vi "CR test.vi"() -> ()   [LabVIEW 2021]
uses:
  Data Model/ELAN Data Model/Type Definitions/Value full.ctl
  Data Unit/ELAN PC Data Unit/Elan units.ctl
  Data Unit/ELAN PC Data Unit/Elan measured variable.ctl
  Data Unit/ELAN PC Data Unit/Elan channel state.ctl
  enums/main_prog_state.ctl
  enums/init_state.ctl
  Master CR.lvclass
  Param/TCP Param/TCP Param.lvclass
  D:/my_projects/projects/Algorithms/Labview/21/Master CR/Param/Param.lvclass
  Master CR.lvclass/Master CR.ctl
  Param/Param.lvclass/Param.ctl
  Param/TCP Param/TCP Param.lvclass/TCP Param.ctl
  <vilib>/Platform/TimedLoop/XDataNode/timing_clust.ctl
  <vilib>/Platform/TimedLoop/XDataNode/nitl_modes.ctl
  <vilib>/Platform/TimedLoop/XDataNode/wakeup.ctl
  enums/close_state.ctl
  Data/Data Model/Read Data Model.vi
  <vilib>/Platform/TimedLoop/XDataNode/XDataNode.xnode
  Modbus_v121c/Data Model/Device Data Model.lvclass
  <vilib>/Platform/TimedLoop/XDataNode/XDNodeRunTimeDep.lvlib
  enums/Param_MB test.lvlib
  Param/Param.lvclass
  Data Model/ELAN Data Model/ELAN Data Model.lvclass
  Data Unit/ELAN PC Data Unit/ELAN PDU.lvclass
panel:
  out "PM3112":dbl[][](array[numeric])
  out "Values":T1[][](array[typedef]) {"Value"."Value" format="%#_6f"}
  in  "Write":bool
  in  "Read":bool
  out "connects":bool[](array[boolean])
  out "DI":bool[][](array[boolean])
  out "AI":u16[][](array[numeric])
  in  "DO":bool[][](array[boolean])
  in  "AOint":u16[][](array[numeric])
  out "comm error":errorcluster
  out "initialise error":errorcluster
  in  "EP_on":bool
  in  "tick":i64=100 caption="Время цикла основной программы" min=5 max=500 step=1
  in  "stop":bool
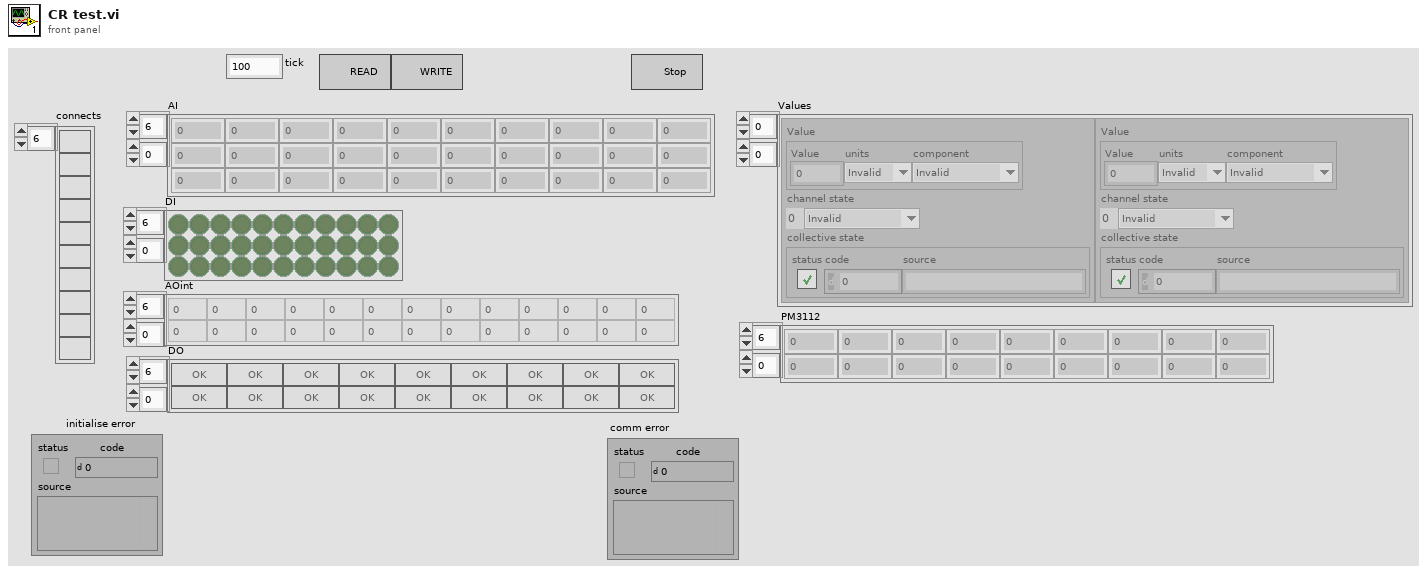
[diagram p1: front panel]
types:
  T1 = typedef "ELAN Data Model.lvclass/Value full.ctl" = cluster{"Value":cluster{"Value":sgl, "units":T2, "component":T3}, "channel state":T4, "collective state":errorcluster}
  T2 = typedef "ELAN PDU.lvclass/Elan units.ctl" = enum16{"Invalid", "no dimension", "ppm", "ppb", "vpm", "ppm C1", "ppm C3", "ppm C6", "mg C/m3", "mg/m3", "%", "% vol", "% of measuring range", "% saturation", "%/°C", "%/K", "% weight", "mV/pH", "mV/mbar", "nA/mbar", "S/m", "S/cm", "mS/m", "mS/cm", "мS/m", "мS/cm", "S", "min", "H", "Pa", "MA", "uV", "MV", "V", "mbar", "hPa", "Ml/min", "kOhm", "MOhm", "S1", "°C", "Hz", "pH", "ug/l", "mg/l", "l/min", "uA", "mg/dm3", "kPa", "kOhm*cm", "MOhm*cm", "°", "1/min", "1/m", "g/m3", "g/l", "% Vol C"}
  T3 = typedef "ELAN PDU.lvclass/Elan measured variable.ctl" = enum16{"Invalid", "no component", "CO", "CO2", "CH4 (Methan)", "C6H14 (Hexan)", "SO2", "NO", "NO2", "CHClF2 (R22)", "C3H8 (Propan)", "C4H10 (Butan)", "O2", "C5H12 (Pentan)", "CnHm (THC)", "P (process pressure)", "pH", "T (temperature)", "C2H4 (Ethen)", "C2H2 (Ethin)", "C3H6 (Propen)", "C4H6", "C4H8", "C2H6", "NH3 (Ammoniak)", "N2O", "C6H6 (Benzol)", "SF6", "CH3OH (Methanol)", "C2H5OH (Ethanol)", "CH2Cl2", "C2H4Cl2", "CH3Cl", "C2H4O", "H2O (water vapor)", "G/l (conductivity)", "C", "S", "N", "CF4", "COCl2 (phosgene)", "CHF3 (R23)", "C2F6 (R116)", "------ (self defined component)", "C2H3Cl", "H2 (Hydrogen)", "Ar", "He", "Cl2", "N2"}
  T4 = typedef "ELAN PDU.lvclass/Elan channel state.ctl" = enum16{"Invalid", "Warm-up", "Pause", "Standby", "Measure", "Zero calibration", "Adjust component slope", "Not yet defined1", "Adjust curve dip", "Adjust linearization sensitivity", "Adjust temperature compensation", "Adjust pressure compensation", "Adjust linearization zero", "Not yet defined2", "Autocal", "Adjust phase", "Zero calibration of O2 sensor", "Synchronous zero calibration", "Purging for synchronous zero calibration", "Adjust analog output", "Adjust analog input", "Autocal check"}
  T5 = cluster{"conn_timeout":i32, "reconn_timeout":i32, "N attempt max":i32, "t_reset_TTL":i32, "write_timeout":i32, "read_timeout":i32, "period":i32}[]
  T6 = cluster{"Remote IP Address":string, "Remote Port":u16}[]
  T7 = typedef "Param_MB test.lvlib/init_state.ctl" = enum16{"Init Data", "Init TMPs", "Init system DB", "Init data DB", "Read Enums", "Init arrays", "Init KFM", "Init Param", "Init AI param", "Init DI param", "Init AO param", "Init DO param", "Init ALR param", "Init save progs", "Read OPC param", "Init Shared Variables", "Init regulators", "Init heaters", "Init Y defs", "Exit"}
  T8 = typedef "Param_MB test.lvlib/main_prog_state.ctl" = enum16{"Read_AI_Param", "Read_DI_Param", "Read_AO_Param", "Read_DO_Param", "Read_ALR_ON_OFF", "Read_ALR_Param", "Read_Param", "Read_REG_Param", "Timers", "AI", "DI", "SendAItoScada", "SendDItoScada", "Alarms", "SendAItoDB", "SendDItoDB", "SendALRtoDB", "Messages", "Controls", "Control HT1", "QN_control", "QN", "QN_state", "Control EB3", "Outputs", "Exit"}
  T9 = cluster{"KFM":string[], "PAR":string[], "AI":string[], "DI":string[], "DI_fast":string[], "AO":string[], "Regs":string[], "DO":string[], "ALR":string[], "System":string[]}
  T10 = cluster{"Enums":cluster{"KFM":string[], "PAR":string[], "AI":string[], "DI":string[], "DI_fast":string[], "AO":string[], "Regs":string[], "DO":string[], "ALR":string[], "System":string[]}, "MBs":refnum<class "Master CR.lvclass">[]}
  T11 = cluster{"current time":timestamp, "Timer_1s":bool, "Timer_10s":bool, "Timer_1day":bool}
  T12 = typedef "XDNodeRunTimeDep.lvlib/timing_clust.ctl" = cluster{"Expected End [f-1]":u64, "Actual End [f-1]":u64, "Finished Late? [f-1]":bool, "Expected End [i-1]":u64, "Actual End [i-1]":u64, "Finished Late? [i-1]":bool, "Expected Start [i]":u64, "Actual Start [i]":u64, "Expected Start [f]":u64, "Actual Start [f]":u64, "Source Name":string, "Structure Name":string, "Period":i64, "Deadline":i64, "Offset":i64, "Start":i64, "Priority":i32, "Timeout":i32, "Mode":T13, "Wakeup Reason":T14, "Error":errorcluster, "Source Type":string, "Secondary Source Type":string, "Global End Time":u64, "Global Start Time":u64, "Frame Duration":u64, "Iteration Duration":u64, "Assigned CPU":i32, "I/O Scan Engine Mode":u32}
  T13 = typedef "XDNodeRunTimeDep.lvlib/nitl_modes.ctl" = enum32{"No Change", "Process missed periods, maintain original phase", "Discard missed periods, maintain original phase", "Process missed periods, ignore original phase", "Discard missed periods, ignore original phase"}
  T14 = typedef "XDNodeRunTimeDep.lvlib/wakeup.ctl" = enum32{"Normal", "Aborted", "Asynchronous wakeup", "Timing source error", "Timed loop error", "Timeout"}
  T15 = typedef "Param_MB test.lvlib/close_state.ctl" = enum16{"QN_state notifier", "QN_control_queue", "ALR notifires", "ALR", "DO notifires", "DO", "AO notifires", "AO", "DI notifres", "DI", "AI notifires", "AI", "OPC", "Param", "SaveMessageProg", "KFM DadaRef", "KFM Registers", "KFM StatusRef", "Exit"}
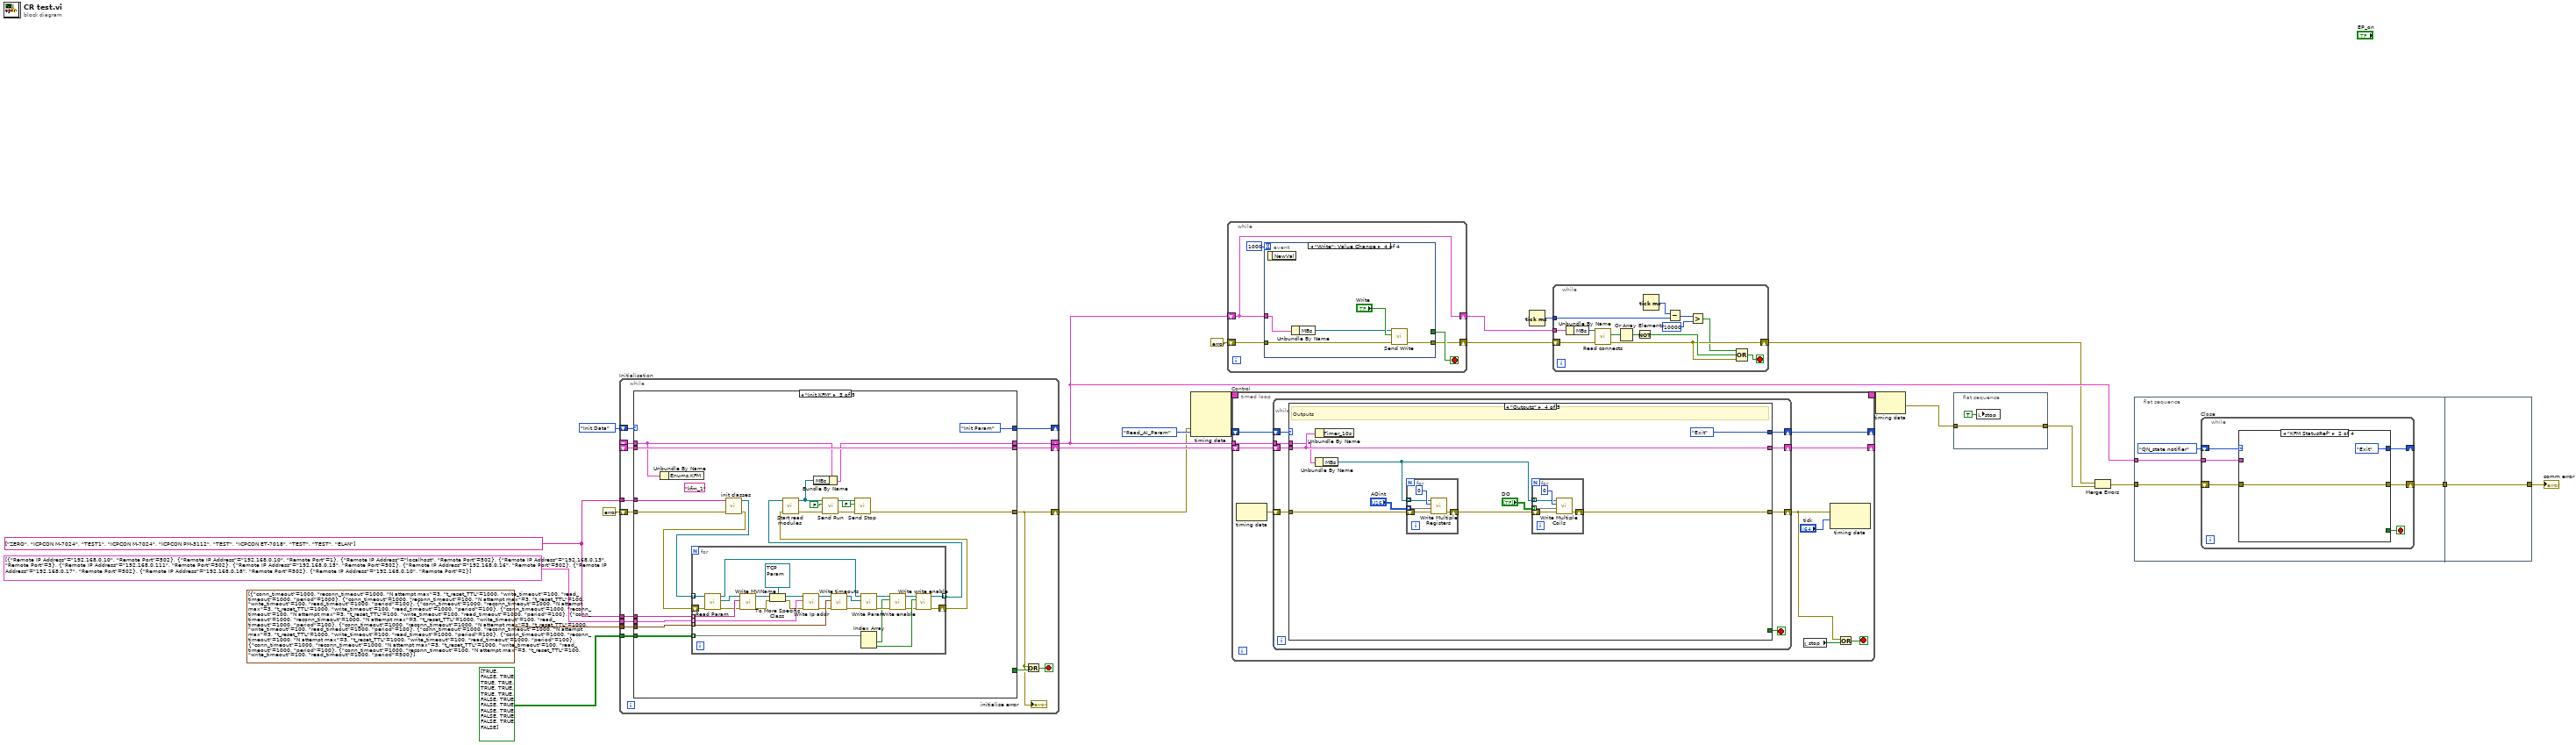
[diagram p0: block diagram]
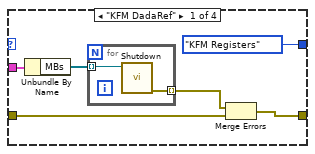
[diagram p2: hidden frame]
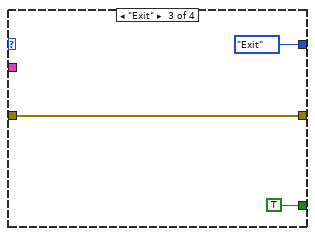
[diagram p3: hidden frame]
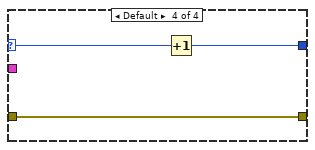
[diagram p4: hidden frame]
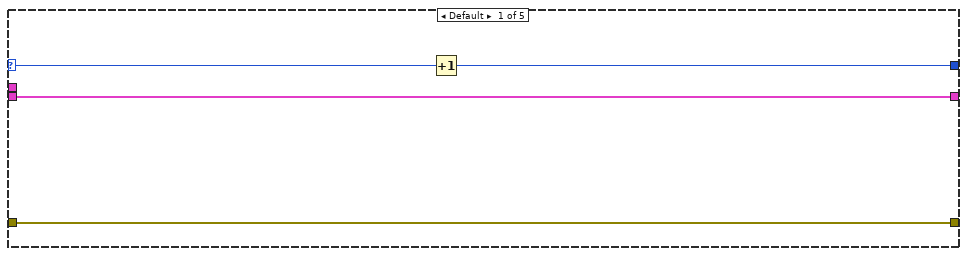
[diagram p5: hidden frame]
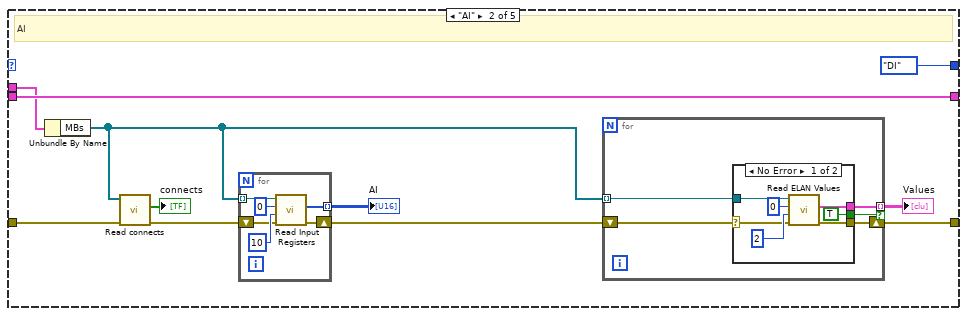
[diagram p6: hidden frame]
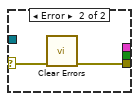
[diagram p7: hidden frame]
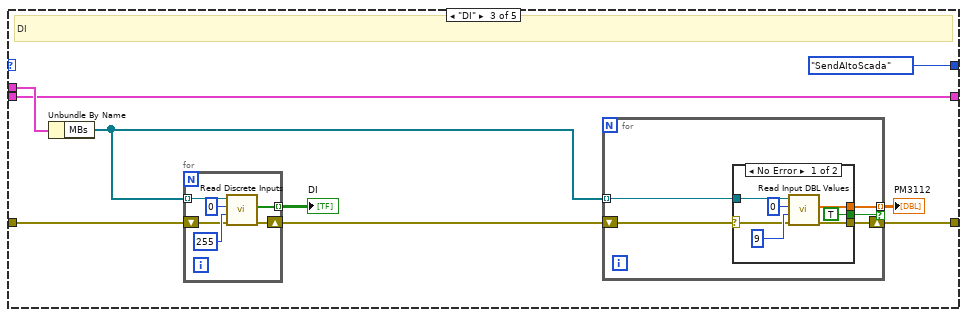
[diagram p8: hidden frame]
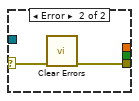
[diagram p9: hidden frame]
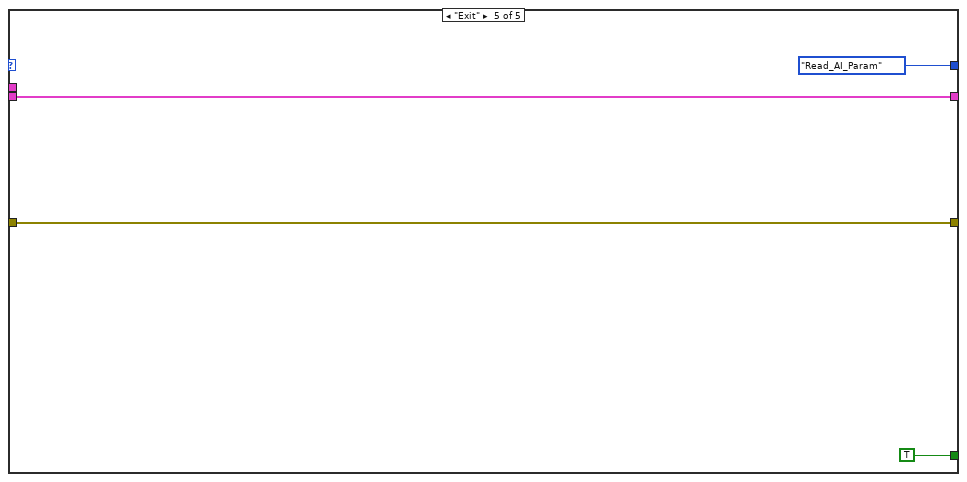
[diagram p10: hidden frame]
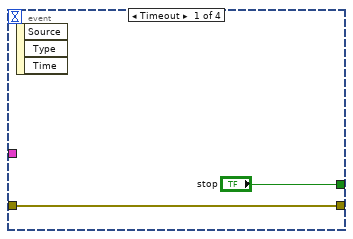
[diagram p11: hidden frame]
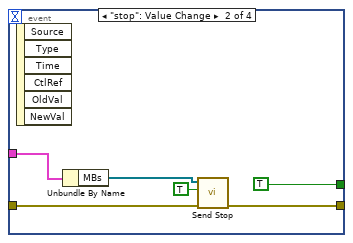
[diagram p12: hidden frame]
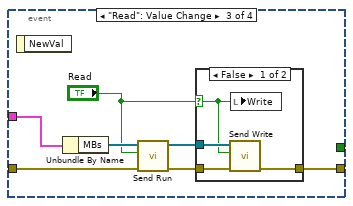
[diagram p13: hidden frame]
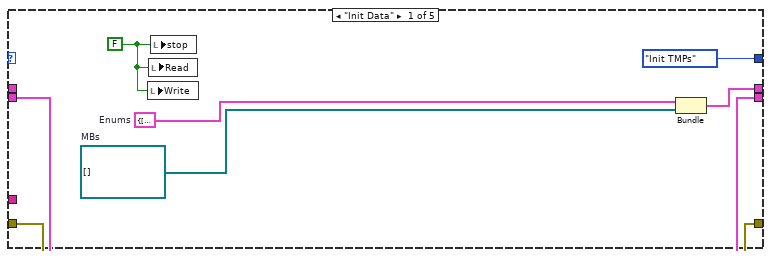
[diagram p15: hidden frame]
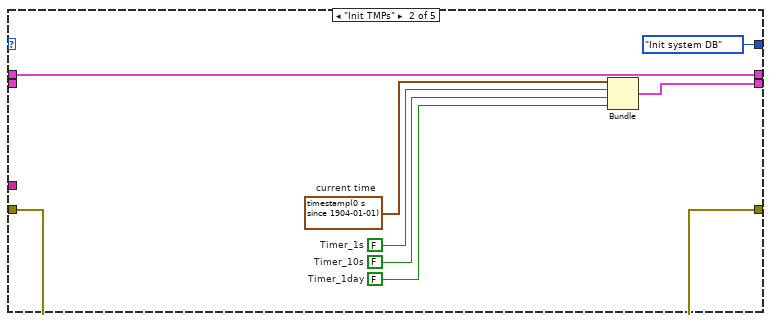
[diagram p16: hidden frame]
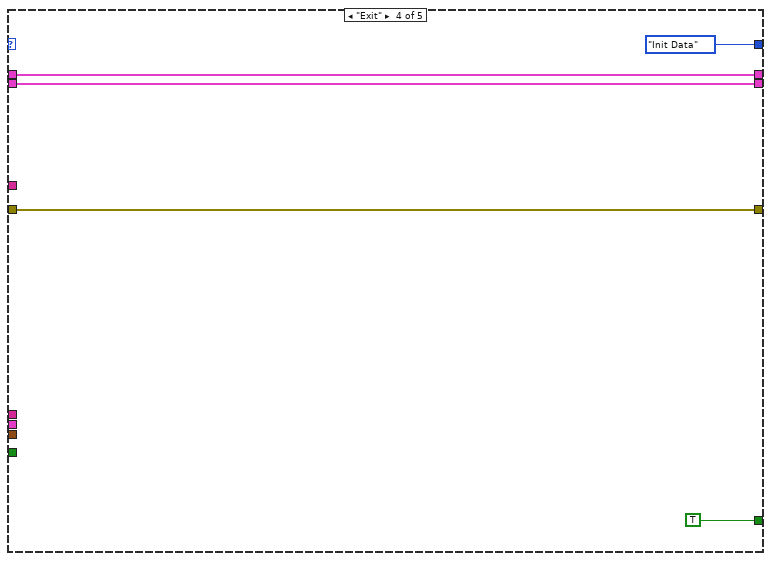
[diagram p17: hidden frame]
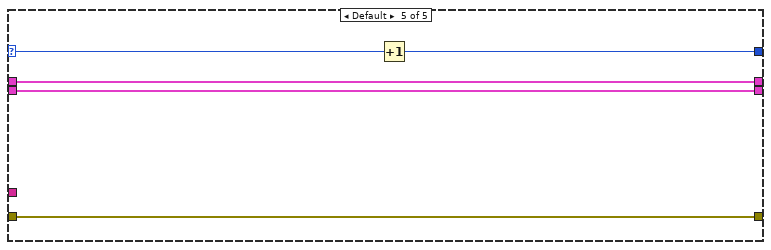
[diagram p18: hidden frame]
diagram:
  w8 = string[] ["ZERO", "ICPCON M-7024", "TEST1", "ICPCON M-7024", "ICPCON PM-3112", "TEST", "ICPCON ET-7018", "TEST", "TEST", "ELAN"] ("MVIName")
  n1 = while "Initialisation" {
    shift-right: [w28] -> w7
    shift-left: errorcluster {"status"=FALSE, "code"=0, "source"=""} ("error out") -> [w34]
    shift-right: [w37] -> w13
    shift-left: _ -> [w35]
    shift-right: [w33] -> _
    shift-left: init_state."Init Data" -> [w36]
    shift-right: [w30] -> w16
    shift-left: _ -> [w29]
    tunnel: w8 -> [w27]
    tunnel: T6 [{"Remote IP Address"="192.168.0.10", "Remote Port"=502}, {"Remote IP Address"="192.168.0.10", "Remote Port"=1}, {"Remote IP Address"="localhost", "Remote Port"=502}, {"Remote IP Address"="192.168.0.13", "Remote Port"=3}, {"Remote IP Address"="192.168.0.111", "Remote Port"=502}, {"Remote IP Address"="192.168.0.15", "Remote Port"=502}, {"Remote IP Address"="192.168.0.16", "Remote Port"=502}, {"Remote IP Address"="192.168.0.17", "Remote Port"=502}, {"Remote IP Address"="192.168.0.18", "Remote Port"=502}, {"Remote IP Address"="192.168.0.10", "Remote Port"=2}] ("IP Address") -> [w26]
    tunnel: T5 [{"conn_timeout"=1000, "reconn_timeout"=1000, "N attempt max"=3, "t_reset_TTL"=1000, "write_timeout"=100, "read_timeout"=1000, "period"=1000}, {"conn_timeout"=1000, "reconn_timeout"=100, "N attempt max"=3, "t_reset_TTL"=100, "write_timeout"=100, "read_timeout"=1000, "period"=100}, {"conn_timeout"=1000, "reconn_timeout"=1000, "N attempt max"=3, "t_reset_TTL"=1000, "write_timeout"=100, "read_timeout"=1000, "period"=100}, {"conn_timeout"=1000, "reconn_timeout"=100, "N attempt max"=3, "t_reset_TTL"=100, "write_timeout"=100, "read_timeout"=1000, "period"=100}, {"conn_timeout"=1000, "reconn_timeout"=1000, "N attempt max"=3, "t_reset_TTL"=1000, "write_timeout"=100, "read_timeout"=1000, "period"=100}, {"conn_timeout"=1000, "reconn_timeout"=1000, "N attempt max"=3, "t_reset_TTL"=1000, "write_timeout"=100, "read_timeout"=1000, "period"=100}, {"conn_timeout"=1000, "reconn_timeout"=1000, "N attempt max"=3, "t_reset_TTL"=1000, "write_timeout"=100, "read_timeout"=1000, "period"=100}, {"conn_timeout"=1000, "reconn_timeout"=1000, "N attempt max"=3, "t_reset_TTL"=1000, "write_timeout"=100, "read_timeout"=1000, "period"=100}, {"conn_timeout"=1000, "reconn_timeout"=1000, "N attempt max"=3, "t_reset_TTL"=1000, "write_timeout"=100, "read_timeout"=1000, "period"=100}, {"conn_timeout"=1000, "reconn_timeout"=100, "N attempt max"=3, "t_reset_TTL"=100, "write_timeout"=100, "read_timeout"=1000, "period"=500}] ("timeouts") -> [w25]
    tunnel: bool[][] [[TRUE, FALSE], [TRUE, TRUE], [TRUE, TRUE], [TRUE, TRUE], [TRUE, FALSE], [TRUE, FALSE], [TRUE, FALSE], [TRUE, FALSE], [TRUE, FALSE], [TRUE, FALSE]] ("enable") -> [w24]
    tunnel: w8 -> [w23]
    stop <- w31 stop-if-true
    # "Initialisation"
    n2 = case shown="\"Init KFM\"" w36 {
      tunnel: [w42 w51 w53 w102 w105] -> w28
      selector: w36 -> [_ _ _ _ w108]
      tunnel: [w43 w50 w54 w103 w106] -> w37
      tunnel: w35 -> [_ w50 w71 w103 w106]
      tunnel: w34 -> [w42 w51 w70 w102 w105]
      tunnel: [init_state."Init TMPs" init_state."Init system DB" init_state."Init Param" init_state."Init Data" w107] -> w33
      tunnel: [_ _ _ TRUE _] -> w32
      tunnel: [w40 w49 w72 w100 w109] -> w30
      tunnel: w29 -> [w40 _ w72 w100 w109]
      tunnel: w27 -> [_ _ w65 _ _]
      tunnel: w26 -> [_ _ w64 _ _]
      tunnel: w25 -> [_ _ w63 _ _]
      tunnel: w24 -> [_ _ w62 _ _]
      tunnel: w23 -> [_ _ w61 _ _]
      frame "Init Data" {
        w38 = FALSE ("stop")
        w39 = refnum<class "Master CR.lvclass">[] []  # MBs
        w41 = T9 {"KFM"=[], "PAR"=[], "AI"=[], "DI"=[], "DI_fast"=[], "AO"=[], "Regs"=[], "DO"=[], "ALR"=[], "System"=[]}  # Enums
        n3 = local write "Write"(w38) -> ()
        n4 = local write "Read"(w38) -> ()
        n5 = local write "stop"(w38) -> ()
        n6 = Bundle("Enums"=w41, "MBs"=w39) -> (w43:T10)  [unwired: 1 in]
      }
      frame "Init TMPs" {
        w45 = FALSE  # Timer_10s
        w46 = FALSE  # Timer_1day
        w47 = FALSE  # Timer_1s
        w48 = timestamp(0 s since 1904-01-01)  # current time
        n7 = Bundle("current time"=w48, "Timer_1s"=w47, "Timer_10s"=w45, "Timer_1day"=w46) -> (w49:T11)  [unwired: 1 in]
      }
      frame "Init KFM" {
        (unwired) "kfm_1" ("KFMTable")
        n8 = Unbundle By Name(w71) -> ()  [unwired: 1 out]
        n9 = call "init classes.vi"("error in (no error)"=w70, "MVINames"=w61) -> ("error out"=w67:errorcluster, "MBs"=w69:refnum<class "Master CR.lvclass">[])  [unwired: 8 in]
        n10 = for {
          tunnel: w69 -> [w75] mode=indexing
          tunnel: w64 -> [w82] mode=indexing
          tunnel: w63 -> [w79] mode=indexing
          tunnel: w65 -> [w97] mode=indexing
          tunnel: w62 -> [w91] mode=indexing
          tunnel: [w87] -> w68 mode=indexing
          shift-right: [w86] -> w66
          shift-left: w67 -> [w99]
          n11 = call "Read Param.vi"("error in (no error)"=w99, "MB_TCP in"=w75) -> ("error out"=w95:errorcluster, "Param"=w74:refnum<class "Param.lvclass">, "MB_TCP out"=w94:refnum<class "Master CR.lvclass">)  [unwired: 7 in]
          n12 = call "Write MVIName.vi"("error in (no error)"=w95, "MVIName"=w97, "MB Param in"=w74) -> ("error out"=w84:errorcluster, "MB Param out"=w96:refnum<class "Param.lvclass">)  [unwired: 7 in]
          n13 = To More Specific Class(target class=refnum<class "TCP Param.lvclass"> refnum ("Param.lvlib:TCP Param.lvclass"), reference=w96, error in=w84) -> (specific class reference=w83:refnum<class "TCP Param.lvclass">, error out=w81:errorcluster)
          n14 = call "Write Ip addr.vi"("error in (no error)"=w81, "IP address"=w82, "MB Param in"=w83) -> ("error out"=w78:errorcluster, "MB Param out"=w80:refnum<class "TCP Param.lvclass">)  [unwired: 7 in]
          n15 = call "Write timeouts.vi"("error in (no error)"=w78, "timeouts"=w79, "MB Param in"=w80) -> ("error out"=w77:errorcluster, "MB Param out"=w76:refnum<class "TCP Param.lvclass">)  [unwired: 7 in]
          n16 = call "Write Param.vi"("error in (no error)"=w77, "Param"=w76, "MB_TCP in"=w94) -> ("error out"=w92:errorcluster, "MB_TCP out"=w93:refnum<class "Master CR.lvclass">)  [unwired: 7 in]
          n17 = Index Array(array=w91) -> (element #1=w90:bool, element #2=w89:bool)  [unwired: 2 in]
          n18 = call "Write enable.vi"("error in (no error)"=w92, "enable"=w90, "Master CR in"=w93) -> ("error out"=w88:errorcluster, "Master CR out"=w98:refnum<class "Master CR.lvclass">)  [unwired: 7 in]
          n19 = call "Write write enable.vi"("error in (no error)"=w88, "write enable"=w89, "Master CR in"=w98) -> ("error out"=w86:errorcluster, "Master CR out"=w87:refnum<class "Master CR.lvclass">)  [unwired: 7 in]
        }
        n20 = call "Start read modules.vi"("error in"=w66, "classes"=w68) -> ("error out"=w56:errorcluster, "classes initialised"=w55:refnum<class "Master CR.lvclass">[])  [unwired: 8 in]
        n21 = Bundle By Name(cluster=w71, "MBs"=w55) -> (w54:T10)
        n22 = call "Send Run.vi"("error in"=w56, "Run"=FALSE, "MCRs"=w55) -> ("error out"=w59:errorcluster, "MCRs out"=w60:refnum<class "Master CR.lvclass">[])  [unwired: 7 in]
        n23 = call "Send Stop.vi"("error in"=w59, "Stop"=FALSE ("Write"), "MCRs"=w60) -> ("error out"=w53:errorcluster)  [unwired: 7 in, 1 out]
      }
      frame "Exit" {
      }
      frame Default {
        n24 = Increment(x=w108) -> (x+1=w107:T7)
      }
    }
    "initialise error" <- w28
    n25 = Or(x=w28, y=w32) -> (x .or. y?=w31:bool)
  }
  n26 = node-c288(w7) -> (w22:T12)  [unwired: 3 in]
  n27 = while {
    shift-right: [w112] -> w4
    shift-left: errorcluster {"status"=FALSE, "code"=0, "source"=""} ("error out") -> [w111]
    shift-right: [w110] -> w3
    shift-left: w13 -> [w110]
    stop <- w113 stop-if-true
    n28 = event shown="[3] \"Write\": Value Change" {
      selector: _ -> [_ _ _ _]
      dyn-events: _ -> [_ _ _ _]
      timeout: 1000 -> [_ _ _ _]
      tunnel: ["stop" TRUE ("stop") _ _] -> w113
      tunnel: w110 -> [_ w117 w129 w139]
      tunnel: w111 -> [w115 w121 w128 w138]
      tunnel: [w115 w120 w123 w137] -> w112
      event Timeout {
        n29 = event-data() -> ()  [unwired: 1 in, 3 out]
      }
      event "stop": Value Change {
        n30 = event-data() -> ()  [unwired: 1 in, 6 out]
        n31 = Unbundle By Name(w117) -> ("MBs"=w118:refnum<class "Master CR.lvclass">[])
        n32 = call "Send Stop.vi"("error in"=w121, "Stop"=TRUE, "MCRs"=w118) -> ("error out"=w120:errorcluster)  [unwired: 7 in, 1 out]
      }
      event "Read": Value Change {
        n33 = event-data() -> ()  [unwired: 1 in, 1 out]
        n34 = Unbundle By Name(w129) -> ("MBs"=w127:refnum<class "Master CR.lvclass">[])
        n35 = call "Send Run.vi"("error in"=w128, "Run"="Read", "MCRs"=w127) -> ("error out"=w125:errorcluster, "MCRs out"=w124:refnum<class "Master CR.lvclass">[])  [unwired: 7 in]
        n36 = case shown="False" "Read" {
          selector: "Read" -> [w131 _]
          tunnel: w125 -> [w133 w134]
          tunnel: w124 -> [w132 _]
          tunnel: [w130 w134] -> w123
          frame False {
            n37 = call "Send Write.vi"("error in"=w133, "Write"=w131, "MCRs"=w132) -> ("error out"=w130:errorcluster)  [unwired: 7 in, 1 out]
            n38 = local write "Write"(w131) -> ()
          }
          frame True {
          }
        }
      }
      event "Write": Value Change {
        n39 = event-data() -> ()  [unwired: 1 in, 1 out]
        n40 = Unbundle By Name(w139) -> ("MBs"=w135:refnum<class "Master CR.lvclass">[])
        n41 = call "Send Write.vi"("error in"=w138, "Write"="Write", "MCRs"=w135) -> ("error out"=w137:errorcluster)  [unwired: 7 in, 1 out]
      }
    }
  }
  n42 = timed-loop "Control" {
    tunnel: w13 -> [w149]
    shift-right: [w147] -> _
    shift-left: w16 -> [w148]
    timing: w22 -> [_]
    timing-out: [_] -> w21
    shift-right: [w145] -> _
    shift-left: main_prog_state."Read_AI_Param" -> [w144]
    stop <- w142 stop-if-true
    n43 = node-c288() -> (w146:errorcluster)  [unwired: 1 in]
    n44 = while {
      tunnel: w149 -> [w157]
      shift-right: [w155] -> w147
      shift-left: w148 -> [w156]
      shift-right: [w150] -> w140
      shift-left: w146 -> [w154]
      shift-right: [w153] -> w145
      shift-left: w144 -> [w152]
      stop <- w151 stop-if-true
      n45 = case shown="\"Outputs\"" w152 {
        tunnel: w154 -> [w158 w171 w198 w227 w241]
        tunnel: w157 -> [_ w164 w200 w228 _]
        tunnel: w156 -> [w160 w170 w199 w229 w242]
        tunnel: [w160 w170 w199 w229 w242] -> w155
        selector: w152 -> [w161 _ _ _ _]
        tunnel: [w159 main_prog_state."DI" main_prog_state."SendAItoScada" main_prog_state."Exit" main_prog_state."Read_AI_Param"] -> w153
        tunnel: [_ _ _ _ TRUE] -> w151
        tunnel: [w158 w169 w195 w223 w241] -> w150
        frame Default {
          n46 = Increment(x=w161) -> (x+1=w159:T8)
        }
        frame "AI" {
          # "AI"
          n47 = Unbundle By Name(w164) -> ("MBs"=w162:refnum<class "Master CR.lvclass">[])
          n48 = call "Read connects.vi"("error in (no error)"=w171, "MCRs in"=w162) -> ("error out"=w166:errorcluster, "connects"=→"connects":bool[])  [unwired: 7 in, 1 out]
          n49 = for {
            tunnel: w162 -> [w174] mode=indexing
            shift-right: [w178] -> w165
            shift-left: w166 -> [w173]
            tunnel: [w175] -> w163 mode=indexing
            n50 = call "Read Input Registers.vi"("error in"=w173, "number of inputs"=u16 10 ("number of coils"), "starting address"=u16 0, "Master CR in"=w174) -> ("error out"=w178:errorcluster, "register values"=w175:u16[])  [unwired: 5 in, 1 out]
          }
          "AI" <- w163
          n51 = for {
            tunnel: w162 -> [w180] mode=indexing
            shift-right: [w183] -> w169
            shift-left: w165 -> [w179]
            tunnel: [w182] -> w167 mode=indexing if=w181
            n52 = case shown="No Error" w179 {
              selector: w179 -> [w185 w192]
              tunnel: [w190 w191] -> w183
              tunnel: [w187 _] -> w182
              tunnel: [TRUE _] -> w181
              tunnel: w180 -> [w184 _]
              frame No Error {
                n53 = call "Read ELAN Values.vi"("error in (no error)"=w185, "number of registers"=u16 2 ("number of coils"), "starting address"=u16 0, "Master CR in"=w184) -> ("error out"=w190:errorcluster, "Values"=w187:T1[])  [unwired: 5 in, 1 out]
              }
              frame Error {
                n54 = call <vilib>:"Clear Errors.vi"("error in (no error)"=w192) -> ("error out"=w191:errorcluster)  [unwired: 5 in, 1 out]
              }
            }
          }
          "Values" <- w167
        }
        frame "DI" {
          # "DI"
          n55 = Unbundle By Name(w200) -> ("MBs"=w194:refnum<class "Master CR.lvclass">[])
          n56 = for {
            tunnel: w194 -> [w217] mode=indexing
            shift-right: [w221] -> w196
            shift-left: w198 -> [w216]
            tunnel: [w218] -> w197 mode=indexing
            n57 = call "Read Discrete Inputs.vi"("error in"=w216, "number of inputs"=u16 255 ("number of coils"), "starting address"=u16 0, "Master CR in"=w217) -> ("error out"=w221:errorcluster, "discrete inputs"=w218:bool[])  [unwired: 5 in, 1 out]
          }
          "DI" <- w197
          n58 = for {
            tunnel: w194 -> [w203] mode=indexing
            shift-right: [w206] -> w195
            shift-left: w196 -> [w202]
            tunnel: [w205] -> w193 mode=indexing if=w204
            n59 = case shown="No Error" w202 {
              selector: w202 -> [w208 w215]
              tunnel: [w213 w214] -> w206
              tunnel: [w210 _] -> w205
              tunnel: [TRUE _] -> w204
              tunnel: w203 -> [w207 _]
              frame No Error {
                n60 = call "Read Input DBL Values.vi"("error in (no error)"=w208, "number of registers"=u16 9 ("number of coils"), "starting address"=u16 0, "Master CR in"=w207) -> ("error out"=w213:errorcluster, "data"=w210:dbl[])  [unwired: 5 in, 1 out]
              }
              frame Error {
                n61 = call <vilib>:"Clear Errors.vi"("error in (no error)"=w215) -> ("error out"=w214:errorcluster)  [unwired: 5 in, 1 out]
              }
            }
          }
          "PM3112" <- w193
        }
        frame "Outputs" {
          # "Outputs"
          n62 = Unbundle By Name(w228) -> ("MBs"=w222:refnum<class "Master CR.lvclass">[])
          n63 = Unbundle By Name(w229) -> ()  [unwired: 1 out]
          n64 = for {
            tunnel: w222 -> [w237] mode=indexing
            shift-right: [w240] -> w224
            shift-left: w227 -> [w236]
            tunnel: "AOint" -> [w238] mode=indexing
            n65 = call-dynamic "Write Multiple Registers.vi"("error in"=w236, "register values"=w238, "starting address"=u16 0, "Master CR in"=w237) -> ("error out"=w240:errorcluster)  [unwired: 6 in, 1 out]
          }
          n66 = for {
            tunnel: w222 -> [w232] mode=indexing
            shift-right: [w235] -> w223
            shift-left: w224 -> [w231]
            tunnel: "DO" -> [w233] mode=indexing
            n67 = call-dynamic "Write Multiple Coils.vi"("error in"=w231, "coils"=w233, "starting address"=u16 0, "Master CR in"=w232) -> ("error out"=w235:errorcluster)  [unwired: 6 in, 1 out]
          }
        }
        frame "Exit" {
        }
      }
    }
    n68 = local read "stop"() -> (w141:bool)
    n69 = node-c288(w140, "tick") -> ()  [unwired: 1 out]
    n70 = Or(x=w140, y=w141) -> (x .or. y?=w142:bool)
  }
  n71 = Tick Count (ms)() -> (millisecond timer value=w2:u32)
  n72 = while {
    shift-right: [w256] -> w1
    shift-left: w4 -> [w263]
    tunnel: w3 -> [w260]
    tunnel: w2 -> [w254]
    stop <- w258 stop-if-true
    n73 = Unbundle By Name(w260) -> ("MBs"=w259:refnum<class "Master CR.lvclass">[])
    n74 = call "Read connects.vi"("error in (no error)"=w263, "MCRs in"=w259) -> ("error out"=w256:errorcluster, "connects"=w262:bool[])  [unwired: 7 in, 1 out]
    n75 = Or Array Elements(Boolean array=w262) -> (logical OR=w261:bool)
    n76 = Not(x=w261) -> (.not. x?=w257:bool)
    n77 = Tick Count (ms)() -> (millisecond timer value=w255:u32)
    n78 = Subtract(x=w255, y=w254) -> (x-y=w253:u32)
    n79 = Greater?(x=w253, y=u32 10000) -> (0:w251:bool)
    n80 = Compound Arithmetic op=OR(w251, w257, w256) -> (w258:bool)
  }
  n81 = node-c288(w21) -> (w6:errorcluster)
  n82 = flat-sequence {
    tunnel: [w264] -> w5
    tunnel: w6 -> [w264]
    frame #0 {
      n83 = local write "stop"(TRUE ("stop")) -> ()
    }
  }
  n84 = Merge Errors(w1, w5) -> (w15:errorcluster)
  n85 = flat-sequence {
    tunnel: w13 -> [w268]
    tunnel: w15 -> [w267]
    tunnel: [w266] -> w14
    tunnel: [w292] -> w19
    tunnel: w14 -> [w292]
    frame #0 {
      n86 = while "Close" {
        shift-right: [w274] -> _
        shift-left: close_state."QN_state notifier" ("Init_state") -> [w275]
        tunnel: w268 -> [w272]
        shift-right: [w270] -> w266
        shift-left: w267 -> [w271]
        stop <- w273 stop-if-true
        n87 = case shown="\"KFM StatusRef\"" w275 {
          selector: w275 -> [_ _ _ w291]
          tunnel: [close_state."KFM Registers" close_state."Exit" close_state."Exit" w290] -> w274
          tunnel: [_ _ TRUE _] -> w273
          tunnel: w272 -> [w281 _ _ _]
          tunnel: w271 -> [w279 w284 w287 w289]
          tunnel: [w278 w284 w287 w289] -> w270
          frame "KFM DadaRef" {
            n88 = Unbundle By Name(w281) -> ("MBs"=w277:refnum<class "Master CR.lvclass">[])
            n89 = for {
              tunnel: w277 -> [w283] mode=indexing
              tunnel: [w282] -> w276 mode=indexing
              n90 = call-dynamic "Shutdown.vi"("MB in"=w283) -> ("error out"=w282:errorcluster)  [unwired: 10 in]
            }
            n91 = Merge Errors(w276, w279) -> (w278:errorcluster)
          }
          frame "KFM StatusRef" {
          }
          frame "Exit" {
          }
          frame Default {
            n92 = Increment(x=w291) -> (x+1=w290:T15)
          }
        }
      }
    }
    frame #1 {
    }
  }
  "comm error" <- w19
